vi "DamnYankeeHindbrainThink.vi"(9 "Queue timeout (ms)":i32=50, 10 "Data queue cluster":T3, 11 "Notifier References":T4) -> ()   [LabVIEW 2013]
doc: "This code takes the raw sensor data being written to the queues from HB sense, filters the data in the queues at need, and sends the data into notifiers that MB and FB can see. If there's nothing in the queue, it times out and nothing is written to the notifiers.\n\nTHIS SHOULD BE RUNNING FASTER THAN HB SENSE, ADJUST TIMOUT VALUES IF THAT IS NOT THE CASE.\n\nEric Schneider, April 2014"
uses:
  Data/TypeDefs/Notifiers.ctl
  Data/TypeDefs/UTM Location.ctl
  Data/TypeDefs/Sail Set Suggestions.ctl
  Data/TypeDefs/Rudder Set Suggestions.ctl
  Data/TypeDefs/OverrideInformation.ctl
  Data/TypeDefs/OverrideMode.ctl
  Data/TypeDefs/MotorSetup.ctl
  Data/TypeDefs/DynamixelSetupInfo.ctl
  Data/TypeDefs/AirmarStatus.ctl
  Data/TypeDefs/HardwareOnline.ctl
  Data/TypeDefs/DynamixelCycleTracker.ctl
  Data/TypeDefs/RC Input Values.ctl
  Classes/Missions/GenericMission/GenericMission.lvclass
  Classes/Waypoint/Waypoint.lvclass
  Data/TypeDefs/GPS-Compass Queue Cluster.ctl
  Data/TypeDefs/WindData Queue Cluster.ctl
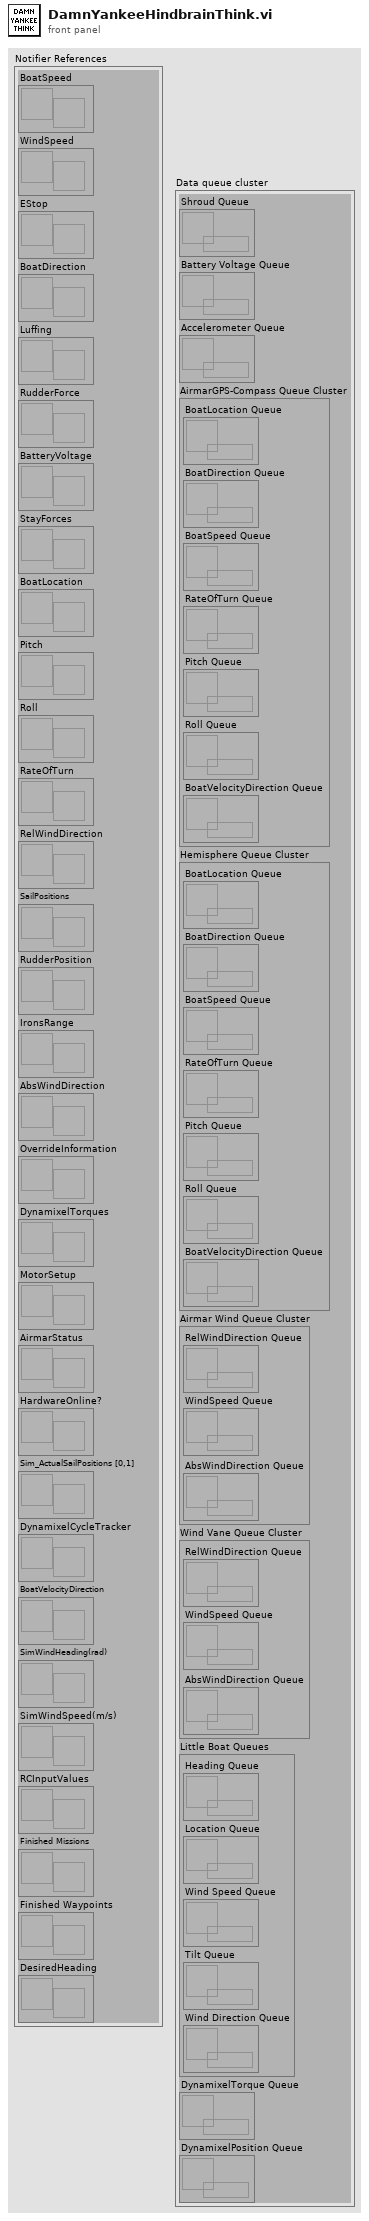
[diagram p1: front panel]
types:
  T1 = typedef "GPS-Compass Queue Cluster.ctl" = cluster{"BoatLocation Queue":refnum<queue>, "BoatDirection Queue":refnum<queue>, "BoatSpeed Queue":refnum<queue>, "RateOfTurn Queue":refnum<queue>, "Pitch Queue":refnum<queue>, "Roll Queue":refnum<queue>, "BoatVelocityDirection Queue ":refnum<queue>}
  T2 = typedef "WindData Queue Cluster.ctl" = cluster{"RelWindDirection Queue":refnum<queue>, "WindSpeed Queue":refnum<queue>, "AbsWindDirection Queue":refnum<queue>}
  T3 = cluster{"Shroud Queue":refnum<queue>, "Battery Voltage Queue":refnum<queue>, "Accelerometer Queue":refnum<queue>, "AirmarGPS-Compass Queue Cluster":T1, "Hemisphere Queue Cluster":T1, "Airmar Wind Queue Cluster":T2, "Wind Vane Queue Cluster":T2, "Little Boat Queues":cluster{"Heading Queue":refnum<queue>, "Location Queue":refnum<queue>, "Wind Speed Queue":refnum<queue>, "Tilt Queue":refnum<queue>, "Wind Direction Queue":refnum<queue>}, "DynamixelTorque Queue":refnum<queue>, "DynamixelPosition Queue":refnum<queue>}
  T4 = typedef "Notifiers.ctl" = cluster{"BoatSpeed":refnum<notifier>, "WindSpeed":refnum<notifier>, "EStop":refnum<notifier>, "BoatDirection":refnum<notifier>, "Luffing":refnum<notifier>, "RudderForce":refnum<notifier>, "BatteryVoltage":refnum<notifier>, "StayForces":refnum<notifier>, "BoatLocation":refnum<notifier>, "Pitch":refnum<notifier>, "Roll":refnum<notifier>, "RateOfTurn":refnum<notifier>, "RelWindDirection":refnum<notifier>, "SailPositions":refnum<notifier>, "RudderPosition":refnum<notifier>, "IronsRange":refnum<notifier>, "AbsWindDirection":refnum<notifier>, "OverrideInformation":refnum<notifier>, "DynamixelTorques":refnum<notifier>, "MotorSetup":refnum<notifier>, "AirmarStatus":refnum<notifier>, "HardwareOnline?":refnum<notifier>, "Sim_ActualSailPositions [0,1]":refnum<notifier>, "DynamixelCycleTracker":refnum<notifier>, "BoatVelocityDirection":refnum<notifier>, "SimWindHeading(rad)":refnum<notifier>, "SimWindSpeed(m/s)":refnum<notifier>, "RCInputValues":refnum<notifier>, "Finished Missions":refnum<notifier>, "Finished Waypoints":refnum<notifier>, "DesiredHeading":refnum<notifier>}
  T5 = typedef "HardwareOnline.ctl" = cluster{"AirmarOnline":bool, "WindvaneOnline":bool, "HemisphereOnline":bool, "StayForceOnline":bool, "BatteryVoltageOnline":bool, "AccelerometerOnline":bool, "MainDynamixel Online":bool, "JibDynamixel Online":bool, "RudderDynamixel Online":bool}
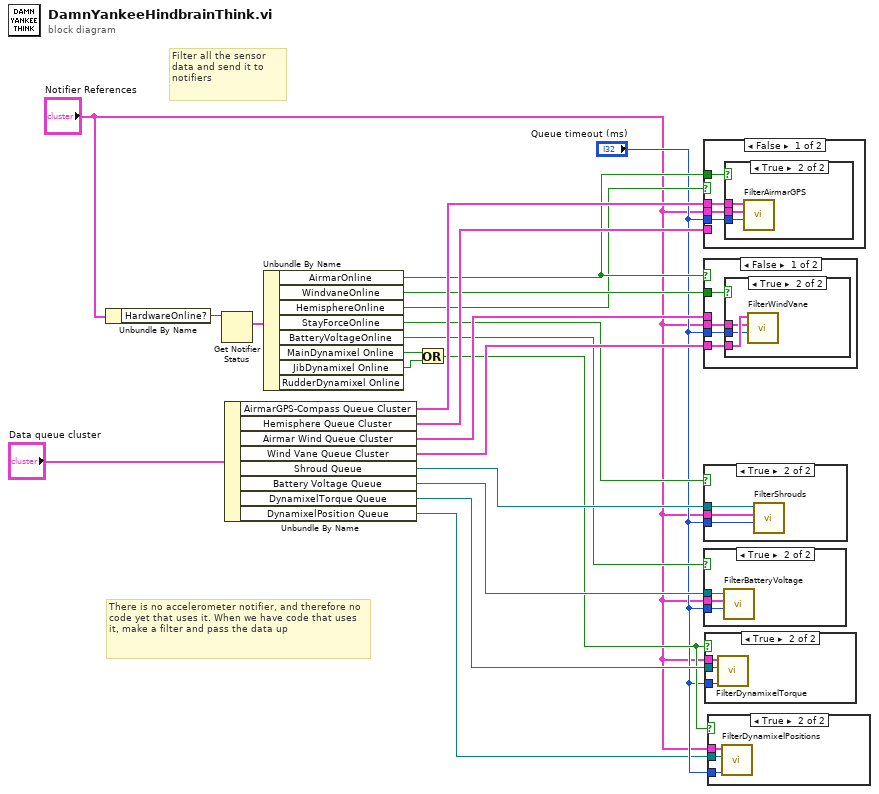
[diagram p0: block diagram]
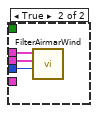
[diagram p5: hidden frame]
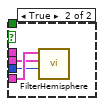
[diagram p7: hidden frame]
diagram:
  # "There is no accelerometer notifier, and therefore no code yet that uses it. When we have code that uses it, make a filter and pass the data up"
  # "Filter all the sensor data and send it to notifiers"
  n1 = Unbundle By Name("Notifier References") -> ("HardwareOnline?"=w17:refnum<notifier>)
  n2 = Get Notifier Status(notifier=w17) -> (current notification=w7:T5)  [unwired: 1 in, 4 out]
  n3 = Unbundle By Name("Data queue cluster") -> ("AirmarGPS-Compass Queue Cluster"=w16:T1, "Hemisphere Queue Cluster"=w18:T1, "Airmar Wind Queue Cluster"=w19:T2, "Wind Vane Queue Cluster"=w15:T2, "Shroud Queue"=w14:refnum<queue>, "Battery Voltage Queue"=w13:refnum<queue>, "DynamixelTorque Queue"=w6:refnum<queue>, "DynamixelPosition Queue"=w3:refnum<queue>)
  n4 = Unbundle By Name(w7) -> ("AirmarOnline"=w11:bool, "WindvaneOnline"=w12:bool, "HemisphereOnline"=w10:bool, "StayForceOnline"=w8:bool, "BatteryVoltageOnline"=w9:bool, "MainDynamixel Online"=w20:bool, "JibDynamixel Online"=w21:bool)  [unwired: 1 out]
  n5 = Or(x=w20, y=w21) -> (x .or. y?=w5:bool)
  n6 = case shown="False" w10 {
    tunnel: w11 -> [w25 _]
    tunnel: "Notifier References" -> [w23 w30]
    tunnel: w16 -> [w24 _]
    tunnel: w18 -> [_ w31]
    tunnel: "Queue timeout (ms)" -> [w22 w29]
    frame False {
      n7 = case shown="True" w25 {
        tunnel: w24 -> [_ w28]
        tunnel: w23 -> [_ w27]
        tunnel: w22 -> [_ w26]
        frame False {
        }
        frame True {
          n8 = call "FilterAirmarGPS.vi"("Queue timeout (ms)"=w26, "NotifierReff"=w27, "AirmarGPS-Compass Queue Cluster"=w28) -> ()  [unwired: 9 in]
        }
      }
    }
    frame True {
      n9 = call "FilterHemisphere.vi"("Queue timeout (ms)"=w29, "NotifierReff"=w30, "Hemisphere Queue Cluster"=w31) -> ()  [unwired: 9 in]
    }
  }
  n10 = case shown="False" w11 {
    tunnel: w12 -> [w35 _]
    tunnel: w15 -> [w34 _]
    tunnel: w19 -> [_ w41]
    tunnel: "Notifier References" -> [w33 w40]
    tunnel: "Queue timeout (ms)" -> [w32 w39]
    frame False {
      n11 = case shown="True" w35 {
        tunnel: w34 -> [_ w38]
        tunnel: w33 -> [_ w37]
        tunnel: w32 -> [_ w36]
        frame False {
        }
        frame True {
          n12 = call "FilterWindVane.vi"("Queue timeout (ms)"=w36, "NotifierReff 2"=w37, "Wind Vane Queue Cluster"=w38) -> ()  [unwired: 9 in]
        }
      }
    }
    frame True {
      n13 = call "FilterAirmarWind.vi"("Queue timeout (ms)"=w39, "NotifierReff"=w40, "Airmar Wind Queue Cluster"=w41) -> ()  [unwired: 9 in]
    }
  }
  n14 = case shown="True" w8 {
    tunnel: w14 -> [_ w44]
    tunnel: "Notifier References" -> [_ w43]
    tunnel: "Queue timeout (ms)" -> [_ w42]
    frame False {
    }
    frame True {
      n15 = call "FilterShrouds.vi"("Queue timeout (ms)"=w42, "NotifierReff 2"=w43, "Queue in"=w44) -> ()  [unwired: 9 in]
    }
  }
  n16 = case shown="True" w9 {
    tunnel: w13 -> [_ w47]
    tunnel: "Notifier References" -> [_ w46]
    tunnel: "Queue timeout (ms)" -> [_ w45]
    frame False {
    }
    frame True {
      n17 = call "FilterBatteryVoltage.vi"("Queue timeout (ms)"=w45, "NotifierReff"=w46, "Queue in"=w47) -> ()  [unwired: 9 in]
    }
  }
  n18 = case shown="True" w5 {
    tunnel: "Queue timeout (ms)" -> [_ w50]
    tunnel: "Notifier References" -> [_ w49]
    tunnel: w6 -> [_ w48]
    frame False {
    }
    frame True {
      n19 = call "FilterDynamixelTorque.vi"("Queue timeout (ms)"=w50, "DynamixelTorque Queue"=w48, "NotifierReff"=w49) -> ()  [unwired: 9 in]
    }
  }
  n20 = case shown="True" w5 {
    tunnel: "Queue timeout (ms)" -> [_ w53]
    tunnel: w3 -> [_ w52]
    tunnel: "Notifier References" -> [_ w51]
    frame False {
    }
    frame True {
      n21 = call "FilterDynamixelPositions.vi"("Queue timeout (ms)"=w53, "DynamixelPosition Queue"=w52, "NotifierReff"=w51) -> ()  [unwired: 9 in]
    }
  }
